vi "Test_ReadValue_NeverWritten_Error.vi"(8 "error in (no error)":errorcluster, 11 "TestCase in":refnum<class "TestValueReferenceTransport.lvclass">) -> (0 "error out":errorcluster, 3 "TestCase out":refnum<class "TestValueReferenceTransport.lvclass">)   [LabVIEW 2017, in "TestValueReferenceTransport.lvclass"]
uses:
  TestValueReferenceTransport.lvclass
  Source/Concrete/ValueReferenceTransport/ValueReferenceTransport.lvclass/ValueReferenceTransport.ctl
  <vilib>/Utility/error.llb/Error Cluster From Error Code.vi
  Source/Concrete/ValueReferenceTransport/ValueReferenceTransport.lvclass
panel:
  out "Return Error":errorcluster
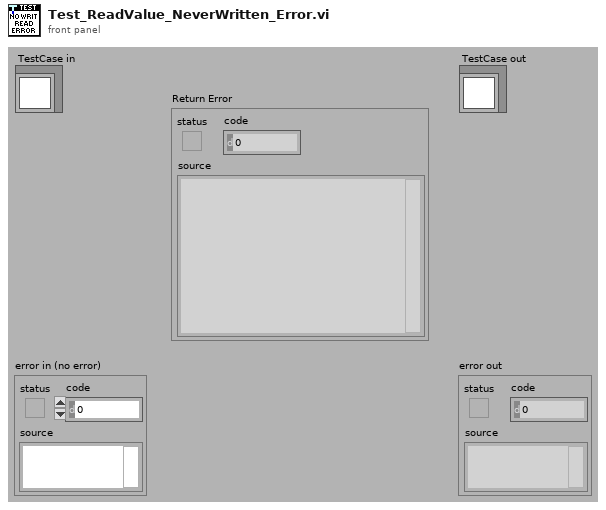
[diagram p1: front panel]
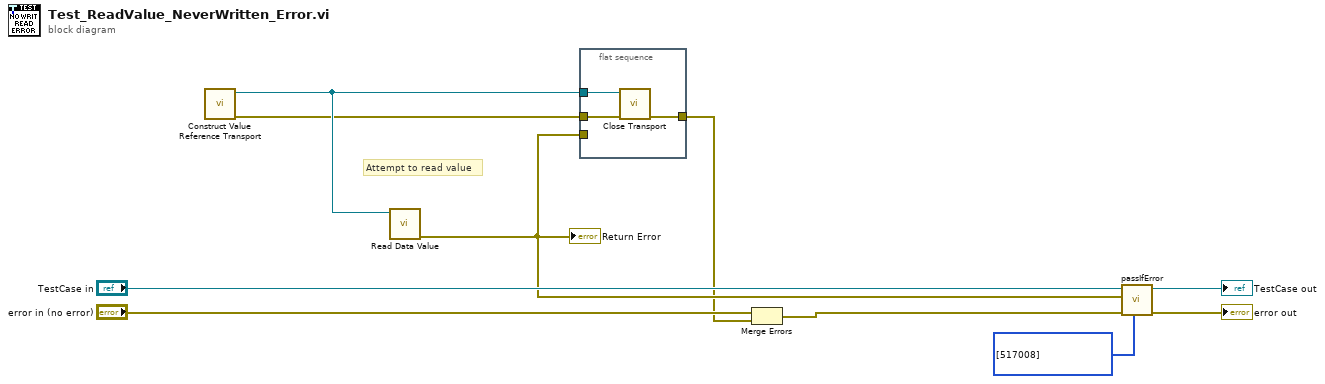
[diagram p0: block diagram]
diagram:
  # "Attempt to read value"
  n1 = call "Construct Value Reference Transport.vi"() -> ("error out"=w3:errorcluster, "ValueReferenceTransport"=w4:refnum<class "ValueReferenceTransport.lvclass">)  [unwired: 10 in]
  n2 = call "Read Data Value.vi"("ValueReferenceTransport In"=w4) -> ("error out"=w2:errorcluster)  [unwired: 8 in, 2 out]
  "Return Error" <- w2
  n3 = flat-sequence {
    tunnel: w4 -> [w13]
    tunnel: w3 -> [w12]
    tunnel: [w11] -> w1
    tunnel: w2 -> [_]
    frame #0 {
      n4 = call-dynamic "Close Transport.vi"("error in (no error)"=w12, "ValueReferenceTransport in"=w13) -> ("error out"=w11:errorcluster)  [unwired: 9 in]
    }
  }
  n5 = Merge Errors("error in (no error)", w1) -> (w5:errorcluster)
  n6 = call-dynamic "passIfError.vi"("passing error codes (default = any error code)"=i32[] [517008], "error in (no error)"=w5, "error"=w2, "TestCase in"="TestCase in") -> ("error out"=→"error out":errorcluster, "TestCase out"=→"TestCase out":refnum<class "TestValueReferenceTransport.lvclass">)  [unwired: 6 in]
